vi "PicAdjust.vi"(1 "Input":dbl[](array[numeric]), 2 "PicAjust":T1={"TranslationVector"=[], "scale"=2.0, "Pitch（x) "=0.0, "Yaw（y)"=0.0, "Roll（z) "=0.0} {"Roll（z)" scale=-90.0..90.0; "Yaw（y)" scale=-90.0..90.0; "Pitch（x)" scale=-90.0..90.0}) -> (0 "子数组":T2=[1.0, 0.0, 0.0, 0.0])   [LabVIEW 2014]
doc: "数据通过四元数法实现图片的调整"
uses:
  <vilib>/robotics/Kinematics/Quaternion.ctl
  <vilib>/robotics/Kinematics/Multiply Quaternion by Quaternion.vi
  <vilib>/robotics/Kinematics/NI_Kinematics.lvlib
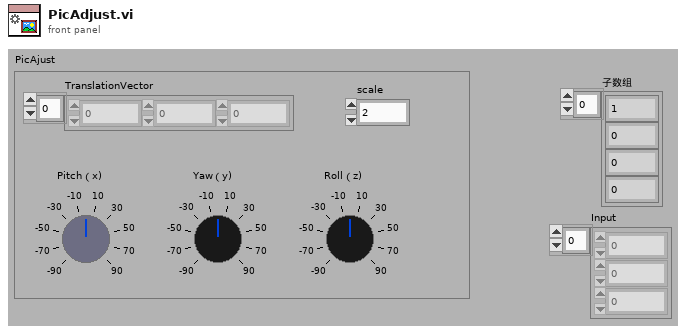
[diagram p1: front panel]
types:
  T1 = cluster{"TranslationVector":dbl[], "scale":dbl, "Pitch（x) ":dbl, "Yaw（y)":dbl, "Roll（z) ":dbl}
  T2 = typedef "NI_Kinematics.lvlib/Quaternion.ctl" = dbl[]
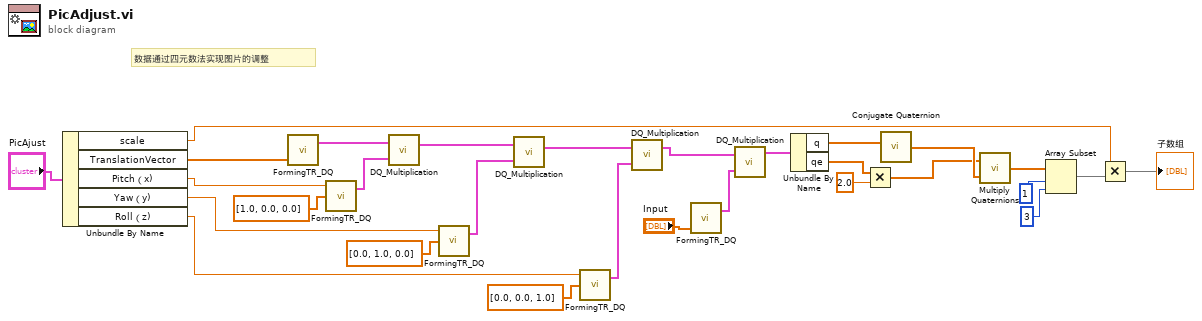
[diagram p0: block diagram]
diagram:
  # "数据通过四元数法实现图片的调整"
  n1 = Unbundle By Name("PicAjust") -> ("scale"=w1:dbl, "TranslationVector"=w3:dbl[], "Pitch（x)"=w6:dbl, "Yaw（y)"=w5:dbl, "Roll（z)"=w4:dbl)
  n2 = call "FormingTR_DQ.vi"("TranslationVector"=w3) -> ("TR_DQ"=w28:cluster{"q":T2, "qe":T2})  [unwired: 2 in, 1 out]
  n3 = call "FormingTR_DQ.vi"("UnitVectorAxis"=dbl[] [1.0, 0.0, 0.0], "Theta(D)"=w6) -> ("TR_DQ"=w21:cluster{"q":T2, "qe":T2})  [unwired: 1 in, 1 out]
  n4 = call "DQ_Multiplication.vi"("DQ2"=w21, "DQ1"=w28) -> ("Product"=w29:cluster{"q":T2, "qe":T2})  [unwired: 1 in]
  n5 = call "FormingTR_DQ.vi"("UnitVectorAxis"=dbl[] [0.0, 1.0, 0.0], "Theta(D)"=w5) -> ("TR_DQ"=w22:cluster{"q":T2, "qe":T2})  [unwired: 1 in, 1 out]
  n6 = call "DQ_Multiplication.vi"("DQ2"=w22, "DQ1"=w29) -> ("Product"=w26:cluster{"q":T2, "qe":T2})  [unwired: 1 in]
  n7 = call "FormingTR_DQ.vi"("UnitVectorAxis"=dbl[] [0.0, 0.0, 1.0], "Theta(D)"=w4) -> ("TR_DQ"=w27:cluster{"q":T2, "qe":T2})  [unwired: 1 in, 1 out]
  n8 = call "DQ_Multiplication.vi"("DQ2"=w27, "DQ1"=w26) -> ("Product"=w9:cluster{"q":T2, "qe":T2})  [unwired: 1 in]
  n9 = call "FormingTR_DQ.vi"("TranslationVector"="Input") -> ("TR_DQ"=w8:cluster{"q":T2, "qe":T2})  [unwired: 2 in, 1 out]
  n10 = call "DQ_Multiplication.vi"("DQ2"=w8, "DQ1"=w9) -> ("Product"=w10:cluster{"q":T2, "qe":T2})  [unwired: 1 in]
  n11 = Unbundle By Name(w10) -> ("q"=w20:T2, "qe"=w14:T2)
  n12 = Multiply(x=w14, y=2.0) -> (x*y=w15:T2)
  n13 = call <vilib>:"Conjugate Quaternion.vi"("quaternion"=w20) -> ("conjugate"=w16:T2)
  n14 = call-poly <vilib>:"Multiply Quaternions.vi"("y"=w16, "quaternion"=w15) -> ("product"=w17:T2)
  n15 = Array Subset(array=w17, index=1 ("索引"), length=3 ("长度")) -> (w2:T2)
  n16 = Multiply(x=w1, y=w2) -> (x*y=→"子数组":T2)
